vi "BRig_Host_recordAnaIn.vi"(5 "input_ai0":i32, 7 "input_ai1":i32, 10 "input_index":i32, 11 "input_dataAnalog":u16[][](array[numeric])) -> (2 "output_index":i32, 3 "output_dataAnalog":u16[][](array[numeric]))   [LabVIEW 2014]
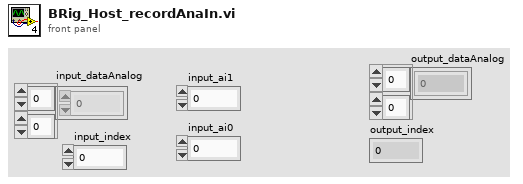
[diagram p1: front panel]
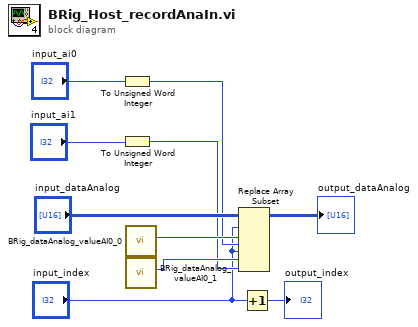
[diagram p0: block diagram]
diagram:
  n1 = To Unsigned Word Integer(number="input_ai0") -> (unsigned 16bit integer=w5:u16)
  n2 = To Unsigned Word Integer(number="input_ai1") -> (unsigned 16bit integer=w4:u16)
  n3 = call "BRig_dataAnalog_valueAI0_0.vi"() -> ("output_valueAI0_0"=w7:i32)  [unwired: 11 in]
  n4 = call "BRig_dataAnalog_valueAI0_1.vi"() -> ("output_valueAI0_1"=w6:i32)  [unwired: 11 in]
  n5 = Replace Array Subset(array="input_dataAnalog", new element #1=w5, index (row) #1="input_index", index (col) #1=w7, new element #2=w4, index (row) #2="input_index", index (col) #2=w6) -> (→"output_dataAnalog":u16[][])
  n6 = Increment(x="input_index") -> (x+1=→"output_index":i32)
